vi "NaN Retries.vi"(8 "error in (no error)":errorcluster, 11 "Optimiser Cell in":refnum<class "Optimiser Cell.lvclass">) -> (0 "error out":errorcluster, 2 "Retry?":bool, 3 "Optimiser Cell out":refnum<class "Optimiser Cell.lvclass">)   [LabVIEW 2020, in "CIRCUS_uServices.lvlib" / "Run Utilities.lvlib" / "Optimiser Cell.lvclass"]
doc: "Increment number of retries after failed calculation of observables"
uses:
  Optimiser Cell.lvclass
  Optimiser Cell.lvclass/Optimiser Cell.ctl
  TALOS/TALOS_PPL.lvlibp
  C:/Users/marco/Documents/GitHub_Lab/CIRCUS/CIRCUS uServices et al/Run Utilities/Cell/Schedule Cell.lvclass
  C:/Users/marco/Documents/GitHub_Lab/CIRCUS/CIRCUS uServices et al/Run Utilities/Optimiser Cell/Optimiser Cell.lvclass
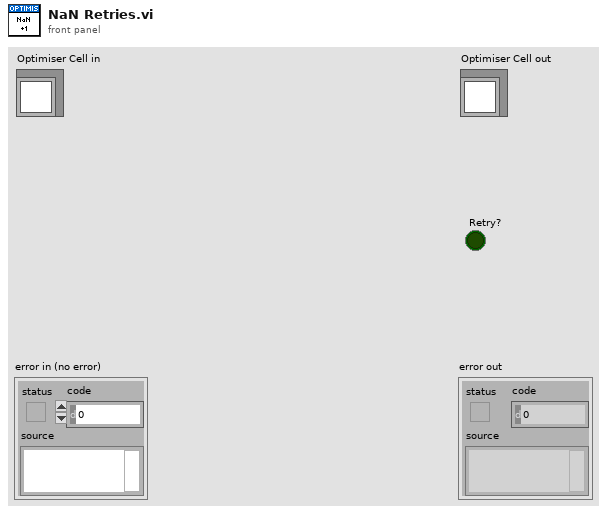
[diagram p1: front panel]
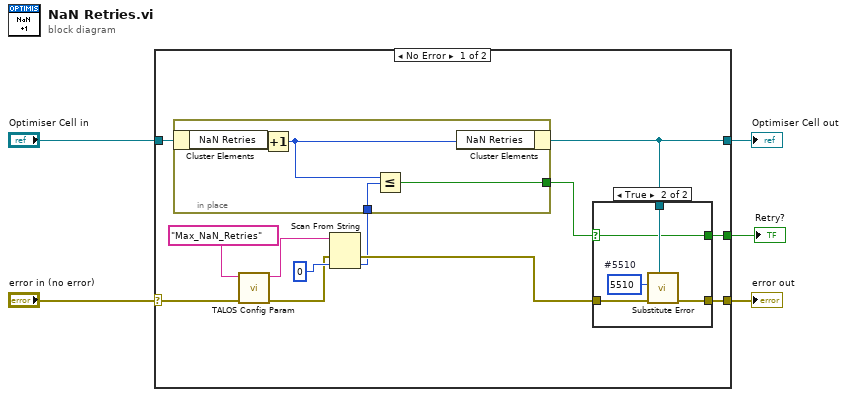
[diagram p0: block diagram]
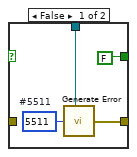
[diagram p2: hidden frame]
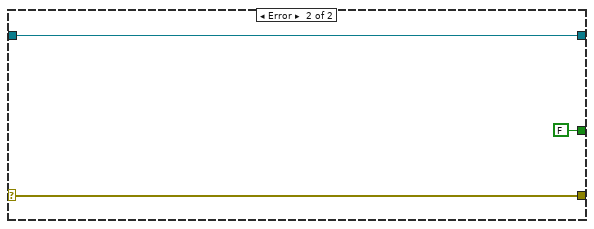
[diagram p3: hidden frame]
diagram:
  n1 = case shown="No Error" "error in (no error)" {
    selector: "error in (no error)" -> [w6 w33]
    tunnel: [w14 w33] -> w4
    tunnel: [w15 w32] -> w2
    tunnel: "Optimiser Cell in" -> [w17 w32]
    tunnel: [w13 FALSE] -> w1
    frame No Error {
      n2 = call "TALOS Config Param.vi"("error in (no error)"=w6, "Parameter Name"="Max_NaN_Retries") -> ("error out"=w7:errorcluster, "Output"=w8:string)  [unwired: 8 in]
      n3 = Scan From String(input string=w8, error in=w7, default 1=u32 0) -> (error out=w12:errorcluster, output 1=w11:u32)  [unwired: 2 in, 2 out]
      n4 = in-place {
        in-place-border: w11 -> [w29]
        in-place-border: [w28] -> w10
        n5 = in-place-cluster #1(w17) -> ("NaN Retries"=w30:u32)
        n6 = Increment(x=w30) -> (x+1=w27:u32)
        n7 = Less Or Equal?(x=w27, y=w29) -> (x <= y?=w28:bool)
        n8 = in-place-cluster #1("NaN Retries"=w27) -> (w15:refnum<class "Optimiser Cell.lvclass">)
      }
      n9 = case shown="True" w10 {
        selector: w10 -> [_ w22]
        tunnel: [w20 w24] -> w14
        tunnel: w15 -> [w19 w23]
        tunnel: [FALSE w22] -> w13
        tunnel: w12 -> [_ w25]
        frame False {
          w21 = 5511  # #5511
          n10 = call "Generate Error.vi"("Class"=w19, "Error Code"=w21) -> ("error out"=w20:errorcluster)  [unwired: 5 in]
        }
        frame True {
          w26 = 5510  # #5510
          n11 = call "Substitute Error.vi"("LabVIEW Object"=w23, "error in (no error)"=w25, "Error Code"=w26) -> ("error out"=w24:errorcluster)  [unwired: 8 in]
        }
      }
    }
    frame Error {
    }
  }
  "error out" <- w4
  "Optimiser Cell out" <- w2
  "Retry?" <- w1
